vi "Verify.vi"(7 "Description":string, 8 "error in (no error)":errorcluster, 10 "Mock":refnum<class "LMock Mock.lvclass">, 11 "LUnit Test Case In":refnum<class "Test Case.lvclass">) -> (0 "error out":errorcluster, 3 "LUnit Test Case Out":refnum<class "Test Case.lvclass">)   [LabVIEW 2020, in "LMock API.lvlib" / "Verifier.lvclass"]
doc: "Verifies that the expected calls have been made to the mock."
uses:
  Verifier.lvclass
  <vilib>/Astemes/LUnit/Test Case.lvclass
  Mock/LMock Mock.lvclass
  <vilib>/Astemes/LUnit/Test Case.lvclass/Test Case.ctl
  <vilib>/Astemes/LUnit/Core/LUnit Test Case/Private/Append Fail Result.vi
  <vilib>/Astemes/LUnit/Core/LUnit Test Case/Private/Append Pass Result.vi
  <vilib>/Astemes/LUnit/Core/LUnit Test Case/Private/Run In UI.vi
  <vilib>/Utility/error.llb/Clear Errors.vi
  Verifier.lvclass/Verifier.ctl
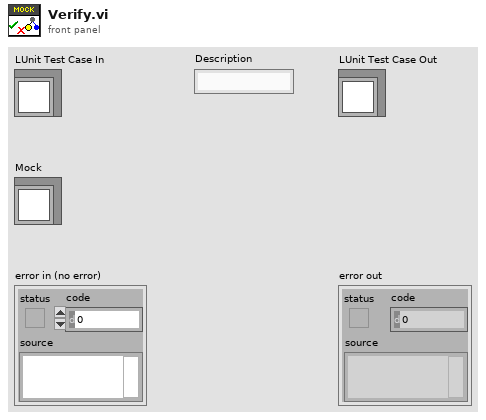
[diagram p1: front panel]
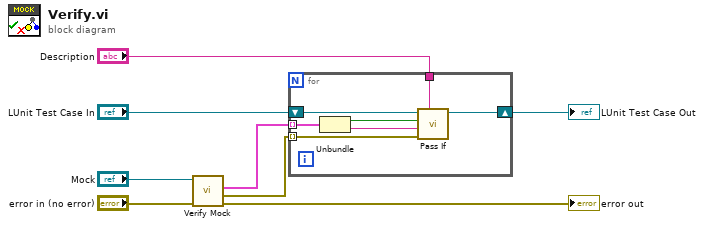
[diagram p0: block diagram]
diagram:
  n1 = call-dynamic "Verify Mock.vi"("error in (no error)"="error in (no error)", "Mock In"="Mock") -> ("error out"=→"error out":errorcluster, "Errors"=w3:errorcluster[], "Results"=w4:cluster{"Passed?":bool, "Message":string}[])  [unwired: 7 in]
  n2 = for {
    shift-right: [w14] -> w7
    shift-left: "LUnit Test Case In" -> [w15]
    tunnel: w4 -> [w12] mode=indexing
    tunnel: w3 -> [w13] mode=indexing
    tunnel: "Description" -> [w9]
    n3 = Unbundle(w12) -> ("Passed?"=w11:bool, "Message"=w10:string)
    n4 = call <vilib>:"Pass If.vi"("Description"=w9, "error in (no error)"=w13, "Message"=w10, "Pass?"=w11, "LUnit Test Case In"=w15) -> ("LUnit Test Case Out"=w14:refnum<class "Test Case.lvclass">)  [unwired: 5 in, 1 out]
  }
  "LUnit Test Case Out" <- w7
